vi "equa.vi"() -> ()   [LabVIEW 2012]
panel:
  in  "Volumen":dbl(slide) scale=0.0..10.0
  in  "Treble":dbl(slide) scale=0.0..10.0
  in  "Voz":dbl(slide) scale=0.0..10.0
  in  "Alto":dbl(slide) scale=0.0..10.0
  in  "Bajo":dbl(slide) scale=0.0..10.0
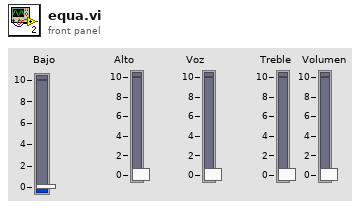
[diagram p1: front panel]
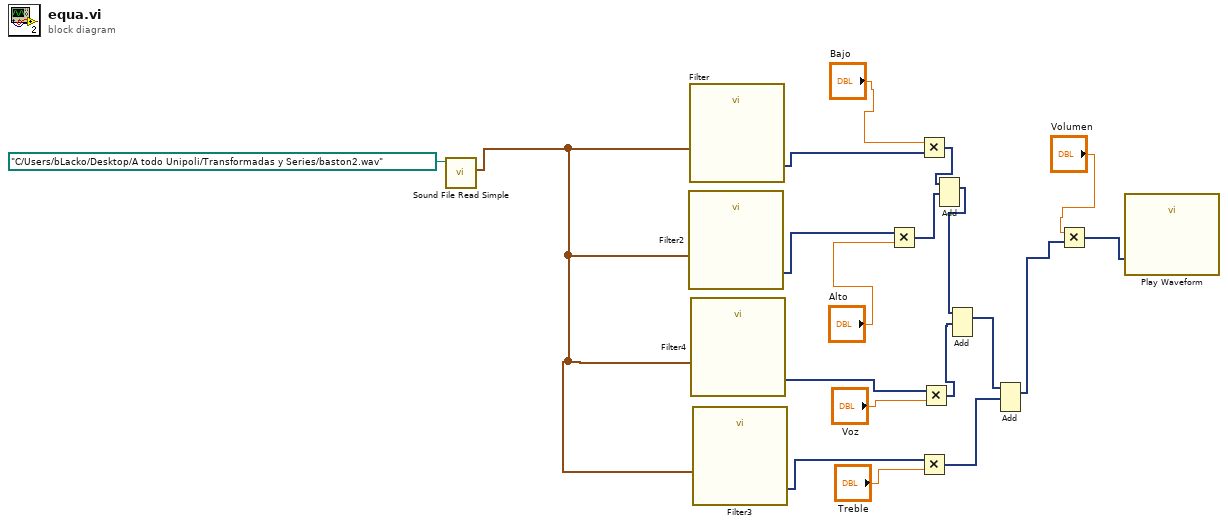
[diagram p0: block diagram]
diagram:
  n1 = call <vilib>:"Sound File Read Simple.vi"("path"=path "C:/Users/bLacko/Desktop/A todo Unipoli/Transformadas y Series/baston2.wav") -> ("data"=w8:waveform(dbl)[])  [unwired: 7 in, 3 out]
  n2 = call "Filter2"("Signal"=w8) -> ("Filtered Signal"=w16:dynamicdata)  [unwired: 9 in, 1 out]
  n3 = call "Filter"("Signal"=w8) -> ("Filtered Signal"=w17:dynamicdata)  [unwired: 9 in, 1 out]
  n4 = call "Filter4"("Signal"=w8) -> ("Filtered Signal"=w12:dynamicdata)  [unwired: 9 in, 1 out]
  n5 = call "Filter3"("Signal"=w8) -> ("Filtered Signal"=w6:dynamicdata)  [unwired: 9 in, 1 out]
  n6 = Multiply(x=w16, y="Alto") -> (x*y=w18:dynamicdata)
  n7 = Multiply(x="Bajo", y=w17) -> (x*y=w19:dynamicdata)
  n8 = Multiply(x=w6, y="Treble") -> (x*y=w5:dynamicdata)
  n9 = Multiply(x=w12, y="Voz") -> (x*y=w10:dynamicdata)
  n10 = Add(1:w18, 2:w19) -> (0:w9:dynamicdata)  [unwired: 1 in, 1 out]
  n11 = Add(1:w10, 2:w9) -> (0:w4:dynamicdata)  [unwired: 1 in, 1 out]
  n12 = Add(1:w5, 2:w4) -> (0:w2:dynamicdata)  [unwired: 1 in, 1 out]
  n13 = Multiply(x="Volumen", y=w2) -> (x*y=w1:dynamicdata)
  n14 = call "Play Waveform"("Data"=w1) -> ()  [unwired: 18 in, 1 out]
